vi "Carbide-Put-AttPercentage.vi"(8 "Error In":errorcluster, 11 "Value":dbl) -> (0 "Error Out":errorcluster)   [LabVIEW 2014]
doc: "André Romero - 2021\nandretec@ifsc.usp.br\nIFSC - USP"
uses:
  Carbide-Global.vi
  <vilib>/httpClient/PUTBuffer.vi
  <vilib>/httpClient/LabVIEWHTTPClient.lvlib
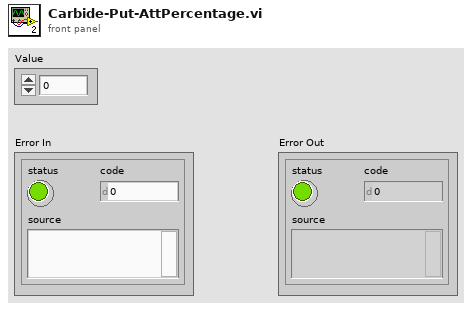
[diagram p1: front panel]
types:
  T1 = typedef "LabVIEWHTTPClient.lvlib/ClientHandle.ctl" = refnum<k1>
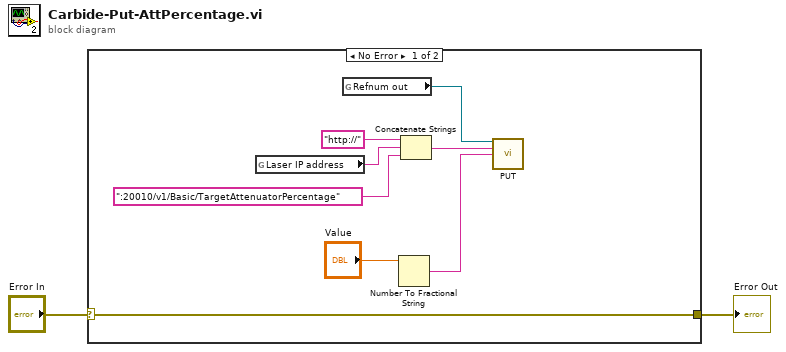
[diagram p0: block diagram]
diagram:
  n1 = case shown="No Error" "Error In" {
    selector: "Error In" -> [w5 w11]
    tunnel: [w5 w11] -> w1
    frame No Error {
      n2 = global read "Carbide-Global.vi" "Laser IP address"() -> (w7:string)
      n3 = global read "Carbide-Global.vi" "Refnum out"() -> (w10:T1)
      n4 = Number To Fractional String(number="Value") -> (F-format string=w3:string)  [unwired: 3 in]
      n5 = Concatenate Strings("http://" ("string"), w7, ":20010/v1/Basic/TargetAttenuatorPercentage" ("string")) -> (w9:string)
      n6 = call-poly <vilib>:"PUT.vi"("client handle"=w10, "url"=w9, "buffer"=w3) -> ()  [unwired: 9 in, 4 out]
    }
    frame Error {
    }
  }
  "Error Out" <- w1
